vi "FindProjectPath.vi"(6 "BuildSpecs? (F)":bool, 8 "error in (no error)":errorcluster, 11 "Library Name":string) -> (0 "error out":errorcluster, 2 "Found?":bool, 3 "Project Path":path)   [LabVIEW 2023, in "CICD.lvlib"]
uses:
  CICD.lvlib
  <userlib>/_OpenG.lib/file/file.llb/openg_file.lvlib
  <vilib>/SLL Toolkit/SLL String/SLL String.lvlib
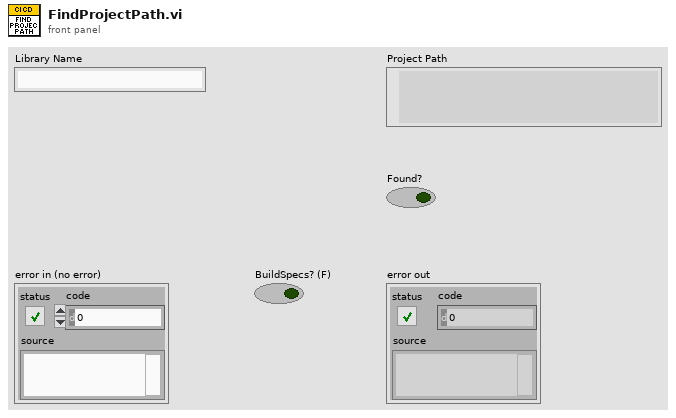
[diagram p1: front panel]
types:
  T1 = typedef "CICD.lvlib/CICDPathConfigs.ctl" = cluster{"GlobalIncludePaths":path[], "GlobalExcludePaths":path[], "BuildSpecsIncludePaths":path[], "ActualDepsIncludePaths":path[], "WorkspacePath":path, "SourceFolderPaths":path[], "ChangedFilesLogpaths":map{string, path}}
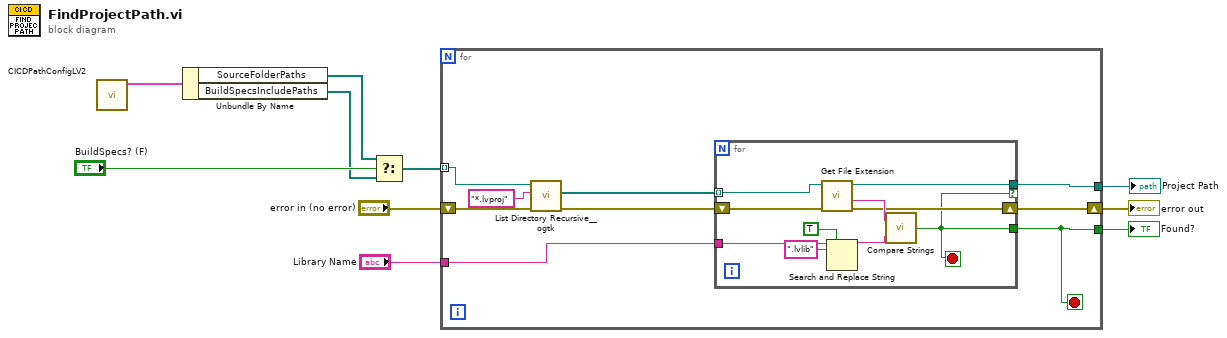
[diagram p0: block diagram]
diagram:
  n1 = call "CICDPathConfigLV2.vi"() -> ("CICD Path Config Out"=w5:T1)  [unwired: 11 in]
  n2 = Unbundle By Name(w5) -> ("SourceFolderPaths"=w2:path[], "BuildSpecsIncludePaths"=w3:path[])
  n3 = Select(t=w2, s="BuildSpecs? (F)", f=w3) -> (s? t:f=w1:path[])
  n4 = for {
    tunnel: [w18] -> w9
    tunnel: [w11] -> w8
    tunnel: "Library Name" -> [w16]
    shift-right: [w13] -> w6
    shift-left: "error in (no error)" -> [w19]
    tunnel: w1 -> [w12] mode=indexing
    stop <- w11 stop-if-true
    n5 = call <userlib>:"List Directory Recursive__ogtk.vi"("error in (no error)"=w19, "pattern"="*.lvproj", "Path"=w12) -> ("error out"=w17:errorcluster, "file paths"=w15:path[])  [unwired: 5 in, 2 out]
    n6 = for {
      tunnel: w15 -> [w28] mode=indexing
      tunnel: w16 -> [w27]
      shift-right: [w22] -> w13
      shift-left: w17 -> [w29]
      tunnel: [w21] -> w18 if=w20
      tunnel: [w20] -> w11
      stop <- w20 stop-if-true
      n7 = call <vilib>:"Get File Extension.vi"("error in (no error)"=w29, "file"=w28) -> ("error out"=w22:errorcluster, "filename without extension"=w24:string, "dup file"=w21:path)  [unwired: 5 in, 2 out]
      n8 = Search and Replace String(replace all?=TRUE ("replace all? (F)"), input string=w27, search string=".lvlib") -> (result string=w23:string)  [unwired: 5 in, 3 out]
      n9 = call <vilib>:"Compare Strings.vi"("y"=w23, "x"=w24) -> ("Equal?"=w20:bool)
    }
  }
  "Project Path" <- w9
  "Found?" <- w8
  "error out" <- w6
